vi "Read File.vi"(8 "error in (no error)":errorcluster, 11 "[Data] Recent User in":refnum<class "[User] Recent Login.lvclass">) -> (0 "error out":errorcluster, 3 "[Data] Recent User out":refnum<class "[User] Recent Login.lvclass">)   [LabVIEW 2020, in "[User] Recent Login.lvclass"]
uses:
  [User] Recent Login.lvclass
  [User] Recent Login.lvclass/[User] Recent Login.ctl
  <vilib>/YU/YU-Encrypt/Base64/Base64.lvclass
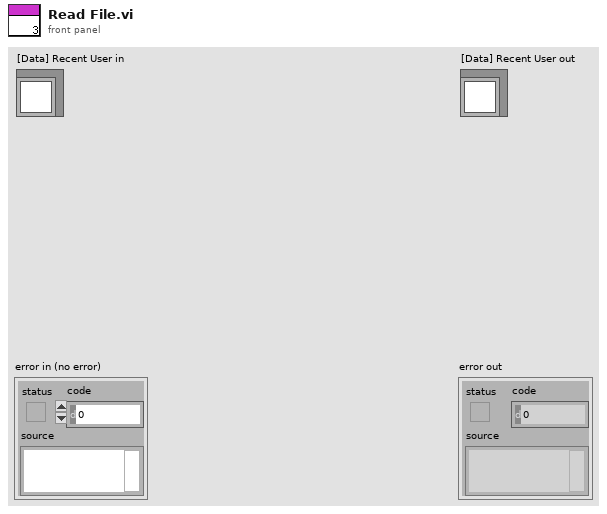
[diagram p1: front panel]
types:
  T1 = enum16{"open", "replace", "create", "open or create", "replace or create", "replace or create with confirmation"}
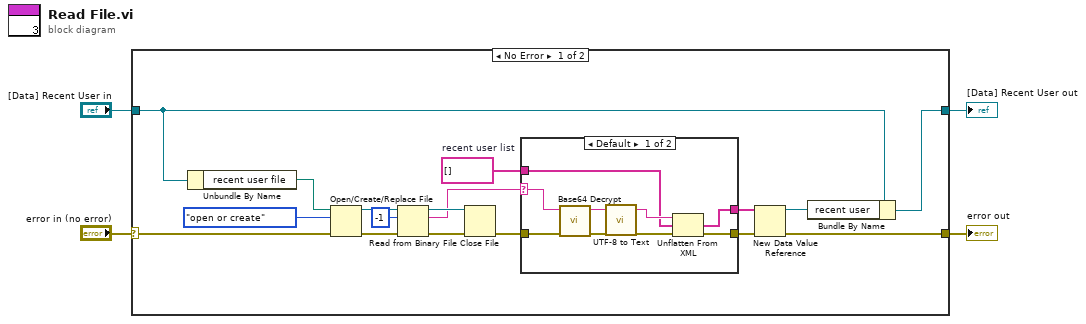
[diagram p0: block diagram]
diagram:
  n1 = case shown="No Error" "error in (no error)" {
    selector: "error in (no error)" -> [w21 w33]
    tunnel: [w7 w33] -> w3
    tunnel: [w8 w32] -> w1
    tunnel: "[Data] Recent User in" -> [w9 w32]
    frame No Error {
      w6 = string[] []  # recent user list
      n2 = Unbundle By Name(w9) -> ("recent user file"=w20:path)
      n3 = Open/Create/Replace File(file path (use dialog)=w20, error in=w21, operation (0:open)=T1."open or create") -> (refnum out=w17:refnum<file>, error out=w18:errorcluster)  [unwired: 3 in, 1 out]
      n4 = Read from Binary File(8:w18, 10:-1 ("count (1)"), 11:w17) -> (0:w15:errorcluster, 2:w13:string, 3:w14:refnum<file>)  [unwired: 3 in, 1 out]
      n5 = Close File(refnum=w14, error in=w15) -> (error out=w12:errorcluster)  [unwired: 1 out]
      n6 = case shown="Default" w13 {
        selector: w13 -> [w28 _]
        tunnel: w12 -> [w29 w31]
        tunnel: [w24 w31] -> w11
        tunnel: [w25 w30] -> w10
        tunnel: w6 -> [w22 w30]
        frame Default {
          n7 = call <vilib>:"Base64 Decrypt.vi"("error in (no error)"=w29, "encrypted data"=w28) -> ("error out"=w26:errorcluster, "data"=w27:string)  [unwired: 8 in]
          n8 = call <vilib>:"UTF-8 to Text.vi"("utf-8 text"=w27) -> ("text"=w23:string)  [unwired: 4 in]
          n9 = Unflatten From XML(xml string=w23, type=w22, error in (no error)=w26) -> (value=w25:string[], error out=w24:errorcluster)
        }
        frame "" {
        }
      }
      n10 = New Data Value Reference(data value=w10, error in=w11) -> (data value reference=w5:refnum<data-value>, error out=w7:errorcluster)
      n11 = Bundle By Name(cluster=w9, "recent user"=w5) -> (w8:refnum<class "[User] Recent Login.lvclass">)
    }
    frame Error {
    }
  }
  "error out" <- w3
  "[Data] Recent User out" <- w1
